vi "echo.vi"(6 "timeout (25000ms)":i32=25000, 8 "error in (no error)":errorcluster, 9 "Target":T1="DDM", 10 "echo byte":u8, 11 "daemon reference in":refnum<k5>) -> (0 "error out":errorcluster, 2 "response":u8, 3 "daemon reference out":refnum<k5>, 5 "command out":string="random")   [LabVIEW 2017]
doc: "<b>Command: </b>\"echo\"\n\n<b>Description: </b> Instructs the target to echo the provided input byte.\n\n<b>Parameters: </b> \n\n 1. Byte to echo (0-255)\n____________________________________________\nDIPC 692 Daemon API 10.0.0.1\nSam Tee - Dyson Technology Ltd\nCopyright (c) 2024, Dyson Technology Ltd"
uses:
  typdef/destination.ctl
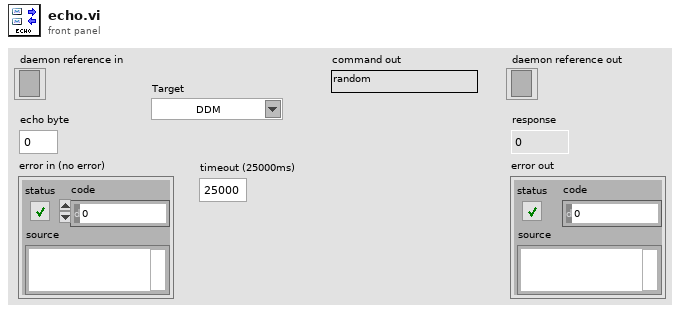
[diagram p1: front panel]
types:
  T1 = typedef "destination.ctl" = string
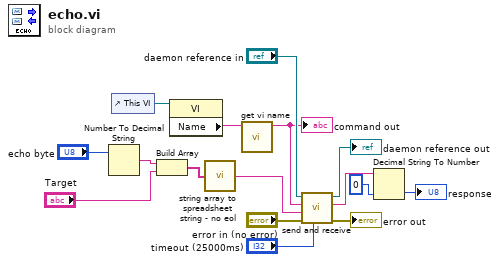
[diagram p0: block diagram]
diagram:
  n1 = Number To Decimal String(number="echo byte") -> (decimal integer string=w4:string)  [unwired: 1 in]
  n2 = control-ref of="This VI"() -> (w7:refnum<vi>)
  n3 = Build Array(w4, "Target") -> (w3:T1[])
  n4 = property class="VI"(reference=w7) -> ("Name"=w6:string)  [unwired: 1 in, 2 out]
  n5 = call "string array to spreadsheet string - no eol.vi"("string array"=w3) -> ("spreadsheet string - no eol"=w2:string)
  n6 = call "get vi name.vi"("library.lvlib:name.vi"=w6) -> ("vi name"=w5:string)  [unwired: 10 in]
  "command out" <- w5
  n7 = call "send and receive.vi"("timeout (25000ms)"="timeout (25000ms)", "error in (no error)"="error in (no error)", "data"=w2, "command"=w5, "daemon reference in"="daemon reference in") -> ("error out"=→"error out":errorcluster, "response"=w11:string, "daemon reference out"=→"daemon reference out":refnum<k5>)  [unwired: 4 in]
  n8 = Decimal String To Number(string=w11, default (0L)=u8 0 ("default (0 I32)")) -> (number=→"response":u8)  [unwired: 1 in, 1 out]
